vi "output.vi"(8 "error in":errorcluster, 10 "data table in":T1, 11 "Daqmx Module runtime in":refnum<class "Daqmx Module runtime.lvclass">) -> (0 "error out":errorcluster, 2 "data table out":T1, 3 "Daqmx Module runtime out":refnum<class "Daqmx Module runtime.lvclass">)   [LabVIEW 2014, in "Daqmx Module runtime.lvclass"]
doc: "Provides an interface for writing data to a module at runtime. While this interface performs no operations, a child should provide an override which may write to any open sessions, references, or interfaces."
uses:
  Daqmx Module runtime.lvclass
  <vilib>/NI/Tag Bus/table/data table.ctl
  Daqmx Module runtime.lvclass/Daqmx Module runtime.ctl
  <vilib>/NI/Tag Bus/table/data polymorphs/read many/read Doubles.vi
  <vilib>/DAQmx/write.llb/DAQmx Write (Analog 1D DBL NChan 1Samp).vi
  <vilib>/NI/Tag Bus/table/data polymorphs/read many/read Booleans.vi
  <vilib>/DAQmx/write.llb/DAQmx Write (Digital 1D Bool NChan 1Samp 1Line).vi
  <vilib>/DAQmx/miscellaneous.llb/DAQmx Fill In Error Info.vi
  <vilib>/NI/Tag Bus/table/data table.lvlib
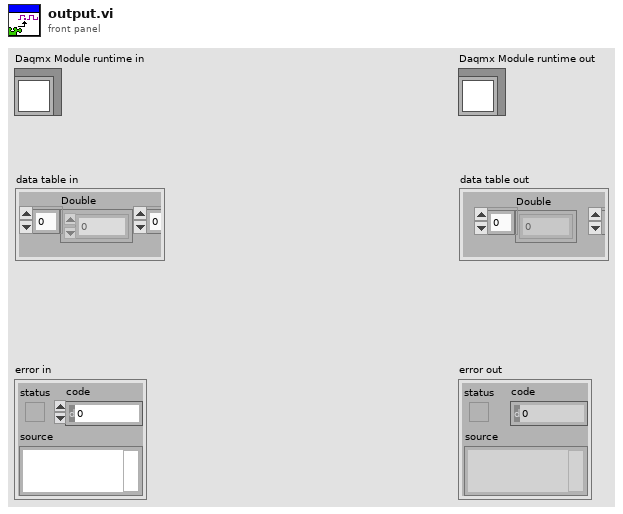
[diagram p1: front panel]
types:
  T1 = typedef "tag bus.lvlib/data table.lvlib/data table.ctl" = cluster{"Double":dbl[], "Single":sgl[], "I64":i64[], "I32":i32[], "I16":i16[], "I8":i8[], "U64":u64[], "U32":u32[], "U16":u16[], "U8":u8[], "Boolean":bool[], "String":string[], "Array of Double":cluster{"DBL Array":dbl[]}[], "Array of Single":cluster{"SGL Array":sgl[]}[], "Array of I64":cluster{"I64 Array":i64[]}[], "Array of I32":cluster{"I32 Array":i32[]}[], "Array of I16":cluster{"I16 Array":i16[]}[], "Array of I8":cluster{"I8 Array":i8[]}[], "Array of U64":cluster{"U64 Array":u64[]}[], "Array of U32":cluster{"U32 Array":u32[]}[], "Array of U16":cluster{"U16 Array":u16[]}[], "Array of U8":cluster{"U8 Array":u8[]}[], "Array of Boolean":cluster{"Boolean Array":bool[]}[], "Array of String":cluster{"String Array":string[]}[]}
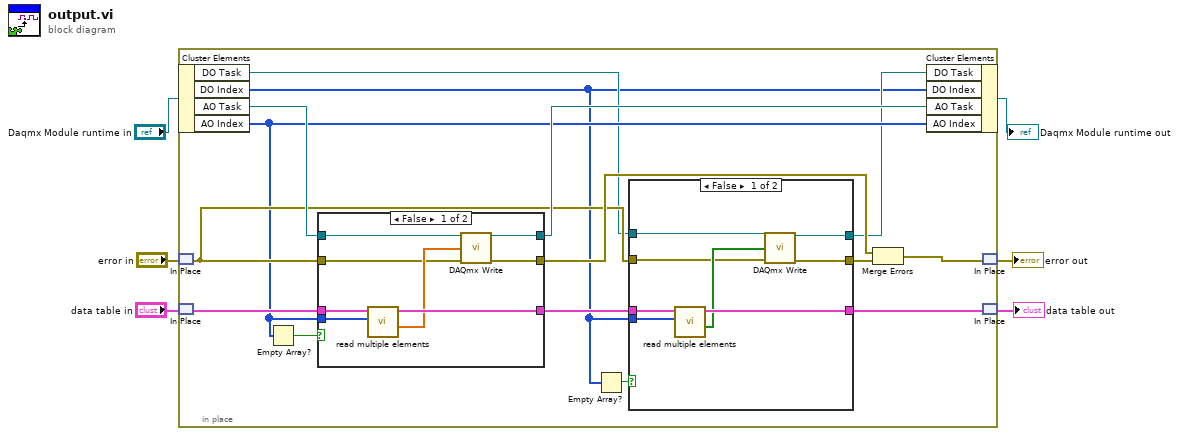
[diagram p0: block diagram]
diagram:
  n1 = in-place {
    n2 = in-place-cluster #1("Daqmx Module runtime in") -> ("DO Task"=w9:refnum<k21>, "DO Index"=w7:i32[], "AO Task"=w20:refnum<k21>, "AO Index"=w11:i32[])
    n3 = in-place-match #2("error in") -> (w13:errorcluster)
    n4 = in-place-match #3("data table in") -> (w21:T1)
    n5 = Empty Array?(array=w11) -> (empty?=w10:bool)
    n6 = case shown="False" w10 {
      tunnel: w21 -> [w40 w42]
      tunnel: [w39 w42] -> w18
      tunnel: w20 -> [w38 w41]
      tunnel: [w37 w41] -> w19
      tunnel: w11 -> [w35 _]
      tunnel: w13 -> [w34 w43]
      tunnel: [w33 w43] -> w16
      frame False {
        n7 = call-poly <vilib>:"read multiple elements.vi"("indices"=w35, "data table in"=w40) -> ("values"=w36:dbl[], "data table out"=w39:T1)  [unwired: 8 in]
        n8 = call-poly <vilib>:"DAQmx Write.vi"("task/channels in"=w38, "data"=w36, "error in"=w34) -> ("task out"=w37:refnum<k21>, "error out"=w33:errorcluster)  [unwired: 10 in, 1 out]
      }
      frame True {
      }
    }
    n9 = Empty Array?(array=w7) -> (empty?=w12:bool)
    n10 = case shown="False" w12 {
      tunnel: w18 -> [w29 w30]
      tunnel: [w28 w30] -> w17
      tunnel: w9 -> [w27 w31]
      tunnel: [w26 w31] -> w8
      tunnel: w7 -> [w24 _]
      tunnel: w13 -> [w23 w32]
      tunnel: [w22 w32] -> w15
      frame False {
        n11 = call-poly <vilib>:"read multiple elements.vi"("indices"=w24, "data table in"=w29) -> ("values"=w25:bool[], "data table out"=w28:T1)  [unwired: 8 in]
        n12 = call-poly <vilib>:"DAQmx Write.vi"("task/channels in"=w27, "data"=w25, "error in"=w23) -> ("task out"=w26:refnum<k21>, "error out"=w22:errorcluster)  [unwired: 10 in, 1 out]
      }
      frame True {
      }
    }
    n13 = Merge Errors(w16, w15) -> (w14:errorcluster)
    n14 = in-place-cluster #1("DO Task"=w8, "DO Index"=w7, "AO Task"=w19, "AO Index"=w11) -> (→"Daqmx Module runtime out":refnum<class "Daqmx Module runtime.lvclass">)
    n15 = in-place-match #2(w14) -> (→"error out":errorcluster)
    n16 = in-place-match #3(w17) -> (→"data table out":T1)
  }
